vi "Initialize.vi"(5 "Transfer Group Status":refnum<class "Status.lvclass">, 6 "FIFO Options":T12, 7 "id":i32, 8 "error in (no error)":errorcluster, 9 "Plugin Buffers":refnum<class "Buffers.lvclass">, 10 "component objects":refnum<class>[](array[class]), 11 "Plugin Configuration":T1={"name"="", "components"=[], "cycle timing"={"priority"=0, "decimation"=1, "offset"=0}, "threads"=[], "Transfer Groups"=[], "settings"=[]} {"Transfer Groups"."Transfers"."channels"."string offset" format="%d bytes"}) -> (0 "error out":errorcluster, 2 "Plugin Threads":refnum<class "Plugin Thread.lvclass">[](array[class]), 3 "Plugin out":refnum<class "Plugin.lvclass">)   [LabVIEW 2017, in "DSF Core.lvlib" / "Plugin.lvclass"]
uses:
  Plugin.lvclass
  Typedefs/DSF FIFO Options.ctl
  Typedefs/DSF Engine Plugin Configuration.ctl
  Typedefs/DSF Timing Info.ctl
  Typedefs/DSF Engine Plugin Thread Configuration.ctl
  Typedefs/DSF Settings Info.ctl
  Typedefs/DSF Engine Transfer Group Configuration.ctl
  Typedefs/DSF Direction.ctl
  Typedefs/DSF Engine Transfer Configuration.ctl
  Typedefs/DSF Byte Order.ctl
  Typedefs/DSF Engine Channel Configuration.ctl
  Typedefs/DSF Data Type.ctl
  Typedefs/DSF Timeout Behavior.ctl
  Buffers/Buffers.lvclass
  Thread/Plugin/Plugin Thread.lvclass
  Transfer Group Status/Status.lvclass
  Plugin.lvclass/Plugin.ctl
  Timing/Timing.lvclass
  DSF Core.lvlib
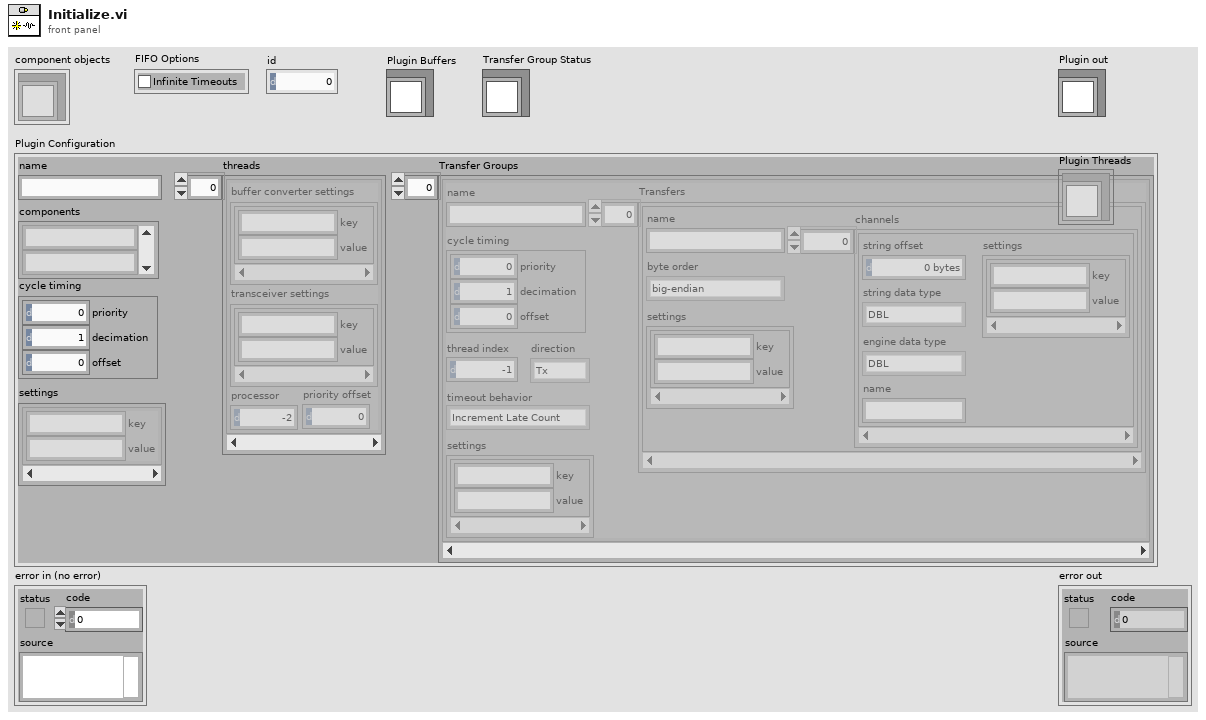
[diagram p1: front panel]
types:
  T1 = typedef "DSF Core.lvlib/DSF Engine Plugin Configuration.ctl" = cluster{"name":string, "components":string[], "cycle timing":T2, "threads":T3[], "Transfer Groups":T5[], "settings":T4}
  T2 = typedef "DSF Core.lvlib/DSF Timing Info.ctl" = cluster{"priority":u64, "decimation":u64, "offset":u64}
  T3 = typedef "DSF Core.lvlib/DSF Engine Plugin Thread Configuration.ctl" = cluster{"buffer converter settings":T4, "transceiver settings":T4, "processor":i32, "priority offset":i16}
  T4 = typedef "DSF Core.lvlib/DSF Settings Info.ctl" = cluster{"key":string, "value":string}[]
  T5 = typedef "DSF Core.lvlib/DSF Engine Transfer Group Configuration.ctl" = cluster{"name":string, "direction":T6, "cycle timing":T2, "thread index":i32, "settings":T4, "Transfers":T7[], "timeout behavior":T11}
  T6 = typedef "DSF Core.lvlib/DSF Direction.ctl" = enum8{"Tx", "Rx"}
  T7 = typedef "DSF Core.lvlib/DSF Engine Transfer Configuration.ctl" = cluster{"name":string, "byte order":T8, "settings":T4, "channels":T9[]}
  T8 = typedef "DSF Core.lvlib/DSF Byte Order.ctl" = enum8{"big-endian", "little-endian"}
  T9 = typedef "DSF Core.lvlib/DSF Engine Channel Configuration.ctl" = cluster{"string offset":u64, "string data type":T10, "engine data type":T10, "name":string, "settings":T4}
  T10 = typedef "DSF Core.lvlib/DSF Data Type.ctl" = enum8{"Bool", "SGL", "DBL", "I8", "I16", "I32", "I64", "U8", "U16", "U32", "U64"}
  T11 = typedef "DSF Core.lvlib/DSF Timeout Behavior.ctl" = enum8{"Increment Late Count", "Throw Error"}
  T12 = typedef "DSF Core.lvlib/DSF FIFO Options.ctl" = cluster{"Infinite Timeouts":bool}
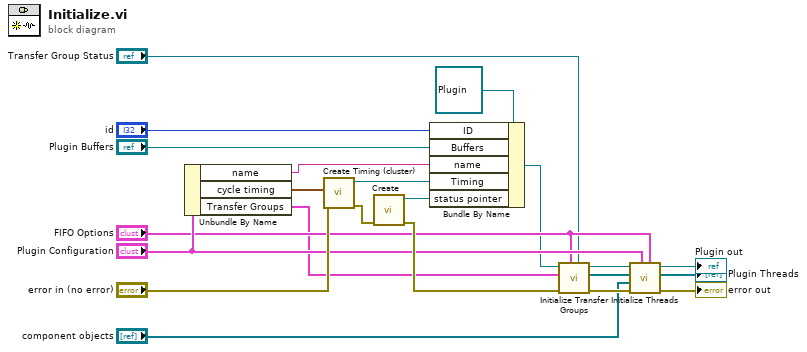
[diagram p0: block diagram]
diagram:
  n1 = Unbundle By Name("Plugin Configuration") -> ("name"=w4:string, "cycle timing"=w18:T2, "Transfer Groups"=w6:T5[])
  n2 = call "Create Timing (cluster).vi"("error in (no error)"="error in (no error)", "cycle timing"=w18) -> ("error out"=w1:errorcluster, "Timing"=w5:refnum<class "Timing.lvclass">)  [unwired: 8 in]
  n3 = call "Create.vi"("error in (no error)"=w1) -> ("error out"=w22:errorcluster, "status pointer"=w2:refnum<class "Status.lvclass">)  [unwired: 9 in]
  n4 = Bundle By Name(cluster=refnum<class "Plugin.lvclass"> refnum ("DSF Core.lvlib:Plugin"), "ID"="id", "Buffers"="Plugin Buffers", "name"=w4, "Timing"=w5, "status pointer"=w2) -> (w7:refnum<class "Plugin.lvclass">)
  n5 = call "Initialize Transfer Groups.vi"("Transfer Group Status"="Transfer Group Status", "FIFO Options"="FIFO Options", "error in (no error)"=w22, "Transfer Group configurations"=w6, "Plugin in"=w7) -> ("error out"=w14:errorcluster, "Transfer Groups"=w9:refnum<class "Transfer Group.lvclass">[], "Plugin out"=w16:refnum<class "Plugin.lvclass">)  [unwired: 4 in]
  n6 = call "Initialize Threads.vi"("FIFO Options"="FIFO Options", "plugin configuration"="Plugin Configuration", "error in (no error)"=w14, "component objects"="component objects", "Transfer Groups"=w9, "Plugin in"=w16) -> ("error out"=→"error out":errorcluster, "Plugin Threads"=→"Plugin Threads":refnum<class "Plugin Thread.lvclass">[], "Plugin out"=→"Plugin out":refnum<class "Plugin.lvclass">)  [unwired: 3 in]
